vi "Close.vi"(8 "error in (no error)":errorcluster, 11 "Camera Config Imaqdx in":refnum<class "Camera Imaqdx CFG.lvclass">) -> (0 "error out":errorcluster, 3 "Camera Config Imaqdx out":refnum<class "Camera Imaqdx CFG.lvclass">)   [LabVIEW 2023, in "Camera Imaqdx CFG.lvclass"]
uses:
  Camera Imaqdx CFG.lvclass
  Camera Imaqdx CFG.lvclass/Camera Imaqdx CFG.ctl
  <vilib>/userDefined/High Color/IMAQdx.ctl
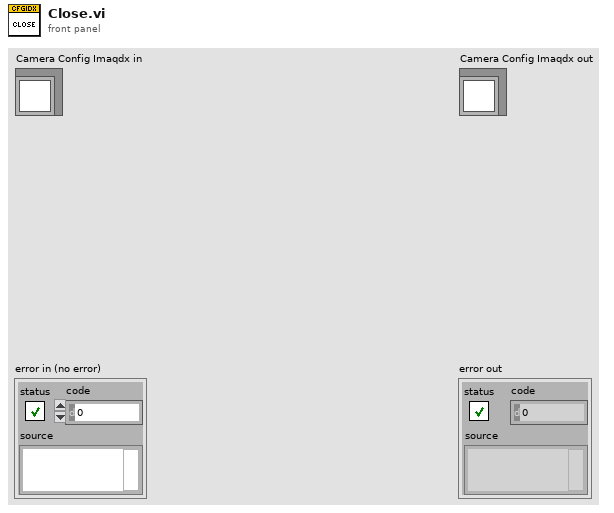
[diagram p1: front panel]
types:
  T1 = typedef "IMAQdx.ctl" = refnum<k21>
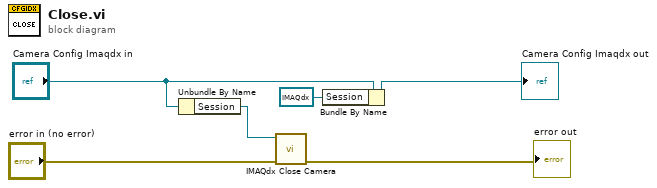
[diagram p0: block diagram]
diagram:
  n1 = Unbundle By Name("Camera Config Imaqdx in") -> ("Session"=w3:T1)
  n2 = call <vilib>:"IMAQdx Close Camera.vi"("error in"="error in (no error)", "Session In"=w3) -> ("error out"=→"error out":errorcluster)  [unwired: 9 in]
  n3 = Bundle By Name(cluster="Camera Config Imaqdx in", "Session"=T1 refnum) -> (→"Camera Config Imaqdx out":refnum<class "Camera Imaqdx CFG.lvclass">)
